vi "MultiplexScanVector.vi"(9 "multiplyer":dbl[](array[numeric]), 11 "initial matrix":dbl[][](array[numeric])) -> (3 "output array":dbl[][](array[numeric]))   [LabVIEW 2018, in "Sequences.lvlib"]
uses:
  Sequences.lvlib
panel:
  out "N line input matrix":i32
  out "N loop":i32
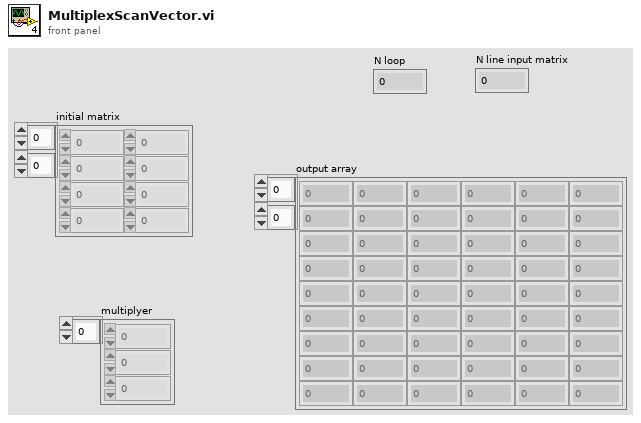
[diagram p1: front panel]
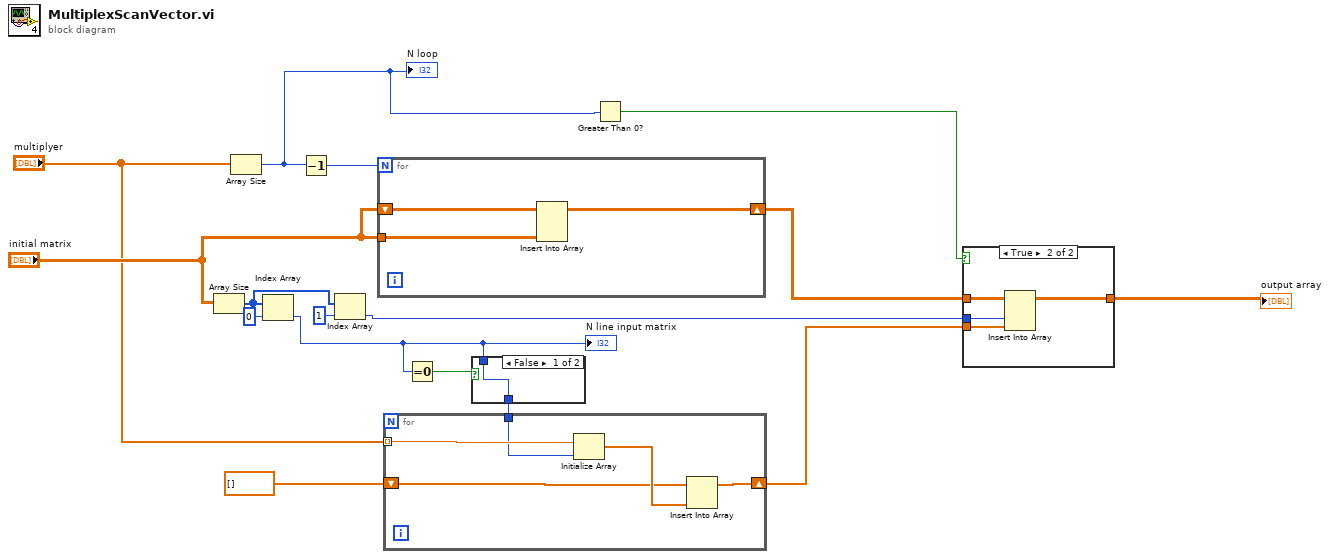
[diagram p0: block diagram]
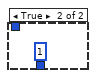
[diagram p2: hidden frame]
diagram:
  n1 = Array Size(array="initial matrix") -> (size(s)=w9:i32[])
  n2 = Array Size(array="multiplyer") -> (size(s)=w5:i32)
  "N loop" <- w5
  n3 = Index Array(array=w9, index=0) -> (element=w1:i32)
  "N line input matrix" <- w1
  n4 = Decrement(x=w5) -> (x-1=w16:i32)
  n5 = Index Array(array=w9, index=1) -> (element=w7:i32)
  n6 = for {
    N: w16 -> [_]
    shift-right: [w19] -> w11
    shift-left: "initial matrix" -> [w18]
    tunnel: "initial matrix" -> [w17]
    n7 = Insert Into Array(array=w18, new element=w17) -> (w19:dbl[][])  [unwired: 2 in]
  }
  n8 = Equal To 0?(x=w1) -> (x = 0?=w3:bool)
  n9 = case shown="False" w3 {
    tunnel: [w20 1 ("dimension size")] -> w2
    tunnel: w1 -> [w20 _]
    frame False {
    }
    frame True {
    }
  }
  n10 = for {
    shift-right: [w23] -> w6
    shift-left: dbl[] [] -> [w24]
    tunnel: "multiplyer" -> [w26] mode=indexing
    tunnel: w2 -> [w22]
    n11 = Initialize Array(w26, w22) -> (w25:dbl[])
    n12 = Insert Into Array(array=w24, new element=w25) -> (w23:dbl[])  [unwired: 1 in]
  }
  n13 = Greater Than 0?(x=w5) -> (x > 0?=w4:bool)
  n14 = case shown="True" w4 {
    tunnel: w11 -> [w27 w31]
    tunnel: [w27 w30] -> w10
    tunnel: w7 -> [_ w28]
    tunnel: w6 -> [_ w29]
    frame False {
    }
    frame True {
      n15 = Insert Into Array(array=w31, index (col)=w28, new element=w29) -> (w30:dbl[][])  [unwired: 1 in]
    }
  }
  "output array" <- w10
